vi "SubVI_Acc_valCheck.vi"(8 "error in (no error)":errorcluster caption="err in", 11 "data":waveform(dbl)[](array[waveform])) -> (0 "error out":errorcluster caption="err out", 3 "val check":bool)   [LabVIEW 2016]
uses:
  <vilib>/measure/mascope.llb/Amplitude and Levels 1 chan.vi
  <vilib>/measure/NI_MAPro.lvlib
panel:
  out "x-y":dbl
  out "Filtered_acc":dynamicdata(graph)=[{"t0"=timestamp(0 s since 1904-01-01), "dt"=1e-05, "Y"=array[2000 elements], "attributes"=variant("NI_ChannelName"=variant(string "필터된"))}]
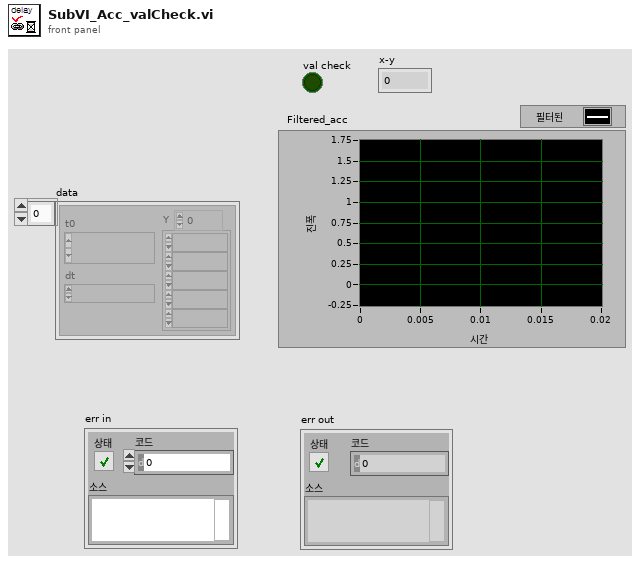
[diagram p1: front panel]
types:
  T1 = cluster{"method":enum32{"histogram", "peak", "auto select"}, "histogram size":i32, "histogram method":enum16{"mode"}, "reserved":dbl}
  T2 = cluster{"Test Information":cluster{"date":string, "custom":string, "oper":string, "package":string, "pkg side":string, "solder":string, "brd side":string, "paste":string, "reflow":string}, "Sensor Set":cluster{"Accelerometer":cluster{"Sensitivity(mV/g)":dbl}, "Strain Guage":cluster{"Ch.":dbl[], "Gage factor":dbl[], "Resistance":dbl[], "Poisson ratio":dbl[]}}, "Resistor Set":cluster{"Criterion Level":dbl, "Res. Set":cluster{"Res. Ch":dbl, "Res. Active":bool, "Res Initial":dbl}[]}, "Test Stop Condition":cluster{"Test cycle":u16, "Fail number in a cycle":u16, "Fail factor":cluster{"Duration":u16, "Fail No.":u16}}, "Acceleration Condition ":cluster{"Shock duration pecent [%]":u16, "Filter cutoff freq":u32}, "Save":cluster{"Save Path":path, "File Name":string}}
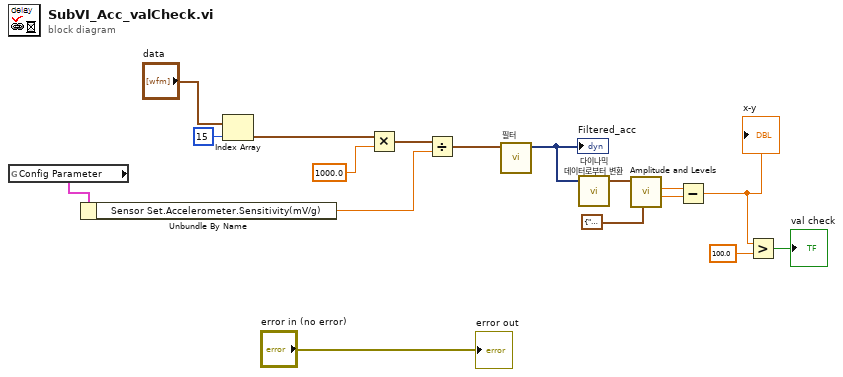
[diagram p0: block diagram]
diagram:
  n1 = global read "글로벌_Config Parameter.vi" "Config Parameter"() -> (w16:T2)
  n2 = Unbundle By Name(w16) -> ("Sensor Set.Accelerometer.Sensitivity(mV/g)"=w13:dbl)
  n3 = Index Array(array="data", index=15 ("인덱스")) -> (element=w2:waveform(dbl))
  n4 = Multiply(x=w2, y=1000.0) -> (x*y=w14:waveform(dbl))
  n5 = Divide(x=w14, y=w13) -> (x/y=w12:waveform(dbl))
  n6 = call "필터"("Signal"=w12) -> ("Filtered Signal"=w17:dynamicdata)  [unwired: 9 in, 1 out]
  "Filtered_acc" <- w17
  n7 = call "다이나믹 데이터로부터 변환"("Dynamic Data Type"=w17) -> ("Waveform"=w11:waveform(dbl))  [unwired: 3 in]
  n8 = call-poly <vilib>:"Amplitude and Levels.vi"("state settings"=T1 {"method"=enum."peak", "histogram size"=256, "histogram method"=enum."mode", "reserved"=1.0}, "signal in"=w11) -> ("low state level"=w9:dbl, "high state level"=w8:dbl)  [unwired: 6 in, 2 out]
  n9 = Subtract(x=w8, y=w9) -> (x-y=w6:dbl)
  "x-y" <- w6
  n10 = Greater?(x=w6, y=100.0) -> (0:→"val check":bool)
  "error out" <- "error in (no error)"
